vi "Table Index Up_End.vi"(7 "Table Index IN":i32, 8 "error in (no error)":errorcluster, 9 "UI Controls Refnum":T3, 10 "Image cluster":T1, 11 "Formatted Table Data":string[][](array[string])) -> (0 "error out":errorcluster, 2 "Table Index OUT":i32, 3 "Saved Image OUT":T2)   [LabVIEW 2012]
uses:
  Custom Control and Typedefs/UI Controls Refnum.ctl
  Custom Control and Typedefs/ChannelSelector_for_PosSave.ctl
  Custom Controls/PositionSaveMod.ctl
  Custom Control and Typedefs/Overlay Control.ctl
  <vilib>/vision/Image Controls.llb/IMAQ Image.ctl
  Custom Control and Typedefs/ImageCluster.ctl
  CommonResource VIs/FormatTableStyle_Commands.ctl
  SubVIs/ImageIO_commands.ctl
panel:
  # "Red (Current Image)"
  # "Green (Saved Image)"
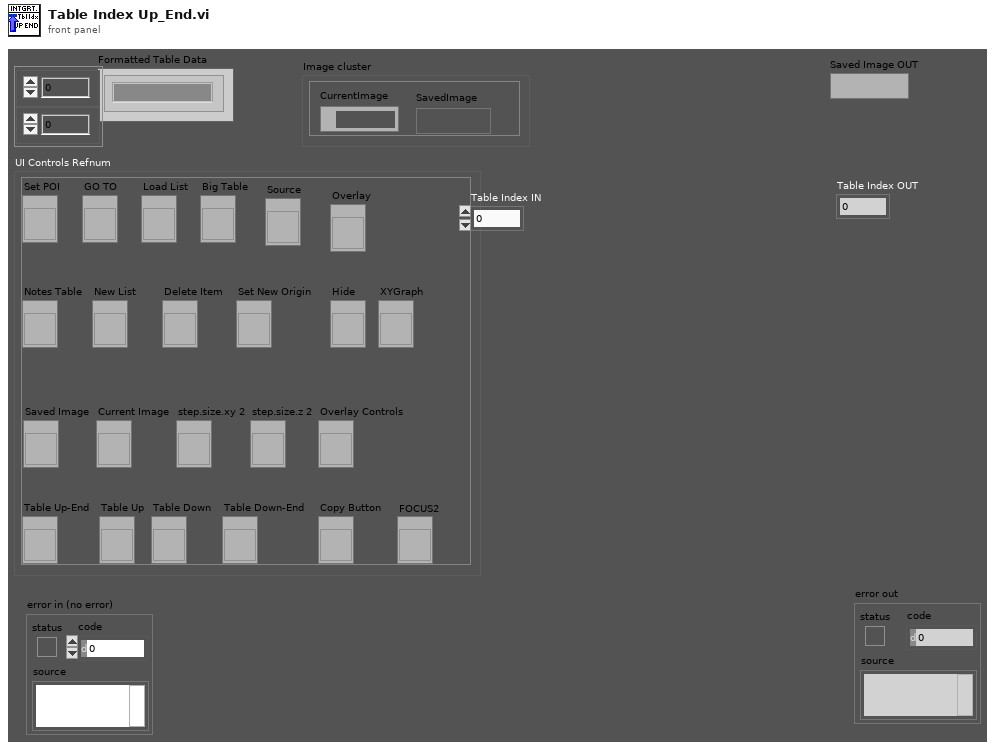
[diagram p1: front panel]
types:
  T1 = typedef "ImageCluster.ctl" = cluster{"CurrentImage":T2, "SavedImage":T2}
  T2 = typedef "IMAQ Image.ctl" = refnum<image>
  T3 = typedef "UI Controls Refnum.ctl" = cluster{"GO TO":refnum<vi>, "Load List":refnum<vi>, "Big Table":refnum<vi>, "Notes Table":refnum<vi>, "New List":refnum<vi>, "Delete Item":refnum<vi>, "Set New Origin":refnum<vi>, "Set POI":refnum<vi>, "Saved Image":refnum<vi>, "Current Image":refnum<vi>, "step.size.xy 2":refnum<vi>, "step.size.z 2":refnum<vi>, "Source":refnum<vi>, "Table Up-End":refnum<vi>, "Table Up":refnum<vi>, "Table Down":refnum<vi>, "Table Down-End":refnum<vi>, "Copy Button":refnum<vi>, "Hide":refnum<vi>, "Overlay Controls":refnum<vi>, "Overlay":refnum<vi>, "XYGraph":refnum<vi>, "FOCUS2":refnum<vi>}
  T4 = typedef "ImageIO_commands.ctl" = enum16{"ReadImage", "WriteImage"}
  T5 = typedef "FormatTableStyle_Commands.ctl" = enum16{"Colour Row", "Uncolour Row", "Bold Row", "Clear table", "UpdateVisibleRows"}
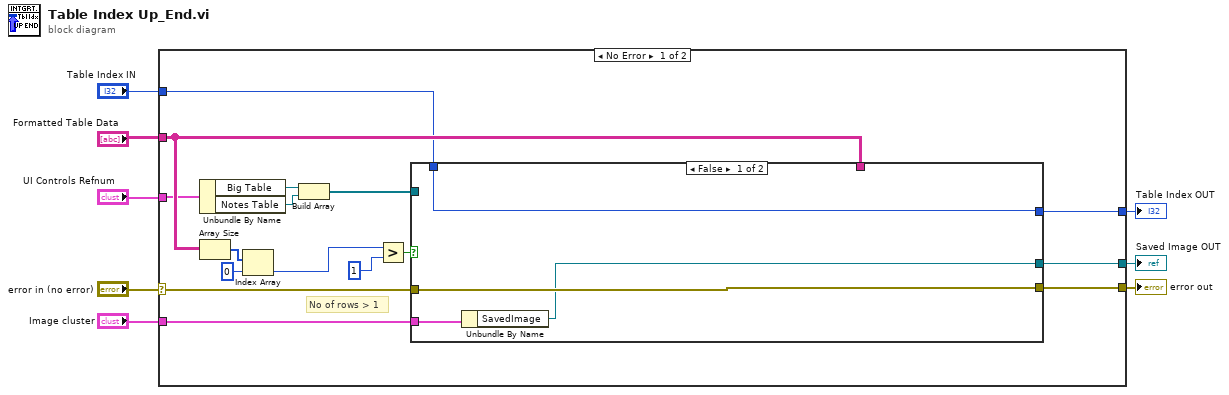
[diagram p0: block diagram]
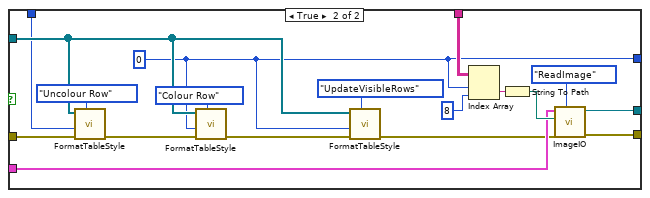
[diagram p2: hidden frame]
diagram:
  n1 = case shown="No Error" "error in (no error)" {
    selector: "error in (no error)" -> [w17 w47]
    tunnel: [w15 w47] -> w8
    tunnel: "Formatted Table Data" -> [w18 _]
    tunnel: "UI Controls Refnum" -> [w16 _]
    tunnel: [w14 _] -> w4
    tunnel: "Image cluster" -> [w13 _]
    tunnel: "Table Index IN" -> [w9 _]
    tunnel: [w12 _] -> w1
    frame No Error {
      # "No of rows > 1"
      n2 = Unbundle By Name(w16) -> ("Big Table"=w23:refnum<vi>, "Notes Table"=w22:refnum<vi>)
      n3 = Array Size(array=w18) -> (size(s)=w20:i32[])
      n4 = Index Array(array=w20, index=0) -> (element=w11:i32)
      n5 = Build Array(w23, w22) -> (w21:refnum<vi>[])
      n6 = Greater?(x=w11, y=1) -> (0:w24:bool)
      n7 = case shown="False" w24 {
        tunnel: [w25 w29] -> w12
        tunnel: w21 -> [_ w40]
        tunnel: w17 -> [w28 w46]
        tunnel: [w28 w32] -> w15
        tunnel: w13 -> [w27 w34]
        tunnel: w18 -> [_ w39]
        tunnel: [w26 w31] -> w14
        tunnel: w9 -> [w25 w30]
        frame False {
          n8 = Unbundle By Name(w27) -> ("SavedImage"=w26:T2)
        }
        frame True {
          w29 = 0 ("y")
          n9 = call "FormatTableStyle.vi"("Format Command"=FormatTableStyle_Commands."Uncolour Row", "Error In"=w46, "Row Index"=w30, "Table reference Array"=w40) -> ("Error Out"=w45:errorcluster)  [unwired: 7 in]
          n10 = call "FormatTableStyle.vi"("Format Command"=FormatTableStyle_Commands."Colour Row", "Error In"=w45, "Row Index"=w29, "Table reference Array"=w40) -> ("Error Out"=w41:errorcluster)  [unwired: 7 in]
          n11 = call "FormatTableStyle.vi"("Format Command"=FormatTableStyle_Commands."UpdateVisibleRows", "Error In"=w41, "Row Index"=w29, "Table reference Array"=w40) -> ("Error Out"=w33:errorcluster)  [unwired: 7 in]
          n12 = Index Array(array=w39, index (row)=w29, index (col)=8 ("disabled index (col)")) -> (element=w37:string)
          n13 = String To Path(string=w37) -> (path=w35:path)
          n14 = call "ImageIO.vi"("Pos_ImageIO_commands"=ImageIO_commands."ReadImage", "Error In"=w33, "Image File Path"=w35, "ImageCluster IN"=w34) -> ("Error Out"=w32:errorcluster, "Saved Image OUT"=w31:T2)  [unwired: 5 in, 1 out]
        }
      }
    }
    frame Error {
    }
  }
  "error out" <- w8
  "Saved Image OUT" <- w4
  "Table Index OUT" <- w1
